vi "VisualizePmuAnalysis.vi"() -> ()   [LabVIEW 2018, in "Visualization.lvlib" / "VisualizeAnalysis.lvclass"]
uses:
  VisualizeAnalysis.lvclass
  <vilib>/event_ctls.llb/usereventprio.ctl
  VisualizeBase/VisualizeBase_class/Requests/clUserEventType.ctl
  <extravilib>/ChannelInstances/Tag-bool/Write With Abort.vi
  <extravilib>/ChannelInstances/Tag-bool/Read With Abort.vi
  <extravilib>/ChannelInstances/Tag-bool/Instantiate.vi
  <vilib>/Utility/error.llb/Error Cluster From Error Code.vi
  <extravilib>/ChannelInstances/Tag-bool/Endpoint.vi
  <vilib>/Utility/file.llb/Read From Spreadsheet File (DBL).vi
  <extravilib>/ChannelInstances/Tag-bool/EndpointRead.vi
  <vilib>/ErrorRing/Error Ring.xnode
  <userlib>/NIST/NISTErrorLib/NISTErrorLib.lvlib
  VisualizeBase/VisualizeBase_class/VisualizeBase.lvclass
  Analysis/AnalysisModule/AnalysisModule.lvlib
  VisualizeSensor/VisualizeSensor.lvclass
  <extravilib>/ChannelInstances/Tag-bool.lvlib
  TestClass/Test.lvclass
panel:
  in  "ModuleID":i32
  in  "btnClearTest":bool
  in  "btnReset":bool
  in  "btnPause":bool
  in  "btnOpen":bool
  in  "btnStop":bool
  in  "PluginName":string="Sensor.RoomAlert1"
  in  "Log Data":bool=TRUE
  out "Data from file":dbl[][](array[numeric])
  out "TVE":cluster{timestamp[], dbl[]}[](graph)
  out "FE":dbl(graph)=1.1347977483922023e-05
  out "ErrorArray":errorcluster[](array[cluster])
  out "RFE":dbl(graph)=-0.0019269131938461162
  out "Data real time":dbl[](array[numeric])
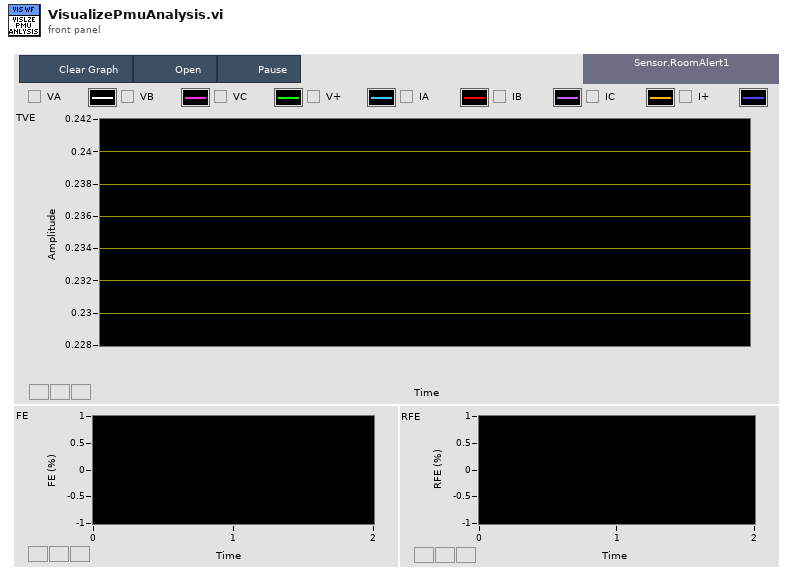
[diagram p1: front panel]
types:
  T1 = typedef "Visualization.lvlib/VisualizeBase.lvclass/clRequestEvents.ctl" = cluster{"StopRequest":refnum<user-event>, "ResetRequest":refnum<user-event>, "FP Pop In or Out":refnum<user-event>}
  T2 = typedef "AnalysisModule.lvlib/clBroadcastEvents.ctl" = cluster{"DidInit":refnum<user-event>, "StatusUpdate":refnum<user-event>, "ErrorReport":refnum<user-event>, "DidStop":refnum<user-event>, "PathToINI":refnum<user-event>, "Config":refnum<user-event>, "ResultReport":refnum<user-event>, "FunctionClass":refnum<user-event>, "State":refnum<user-event>, "FunctionParams":refnum<user-event>, "Duration":refnum<user-event>}
  T3 = enum16{"open", "open or create", "create or replace", "create", "open (read-only)"}
  T4 = typedef "Visualization.lvlib/VisualizeBase.lvclass/clUserEventType.ctl" = cluster{"BusIndex":i8, "Data":variant}
  T5 = typedef "usereventprio.ctl" = enum32{"high priority", "normal priority"}
  T6 = typedef "Tag-bool.lvlib/))Channel.ctl" = refnum<queue>
  T7 = typedef "sizeaction.ctl" = enum32{"Minimized", "Maximized", "Resized"}
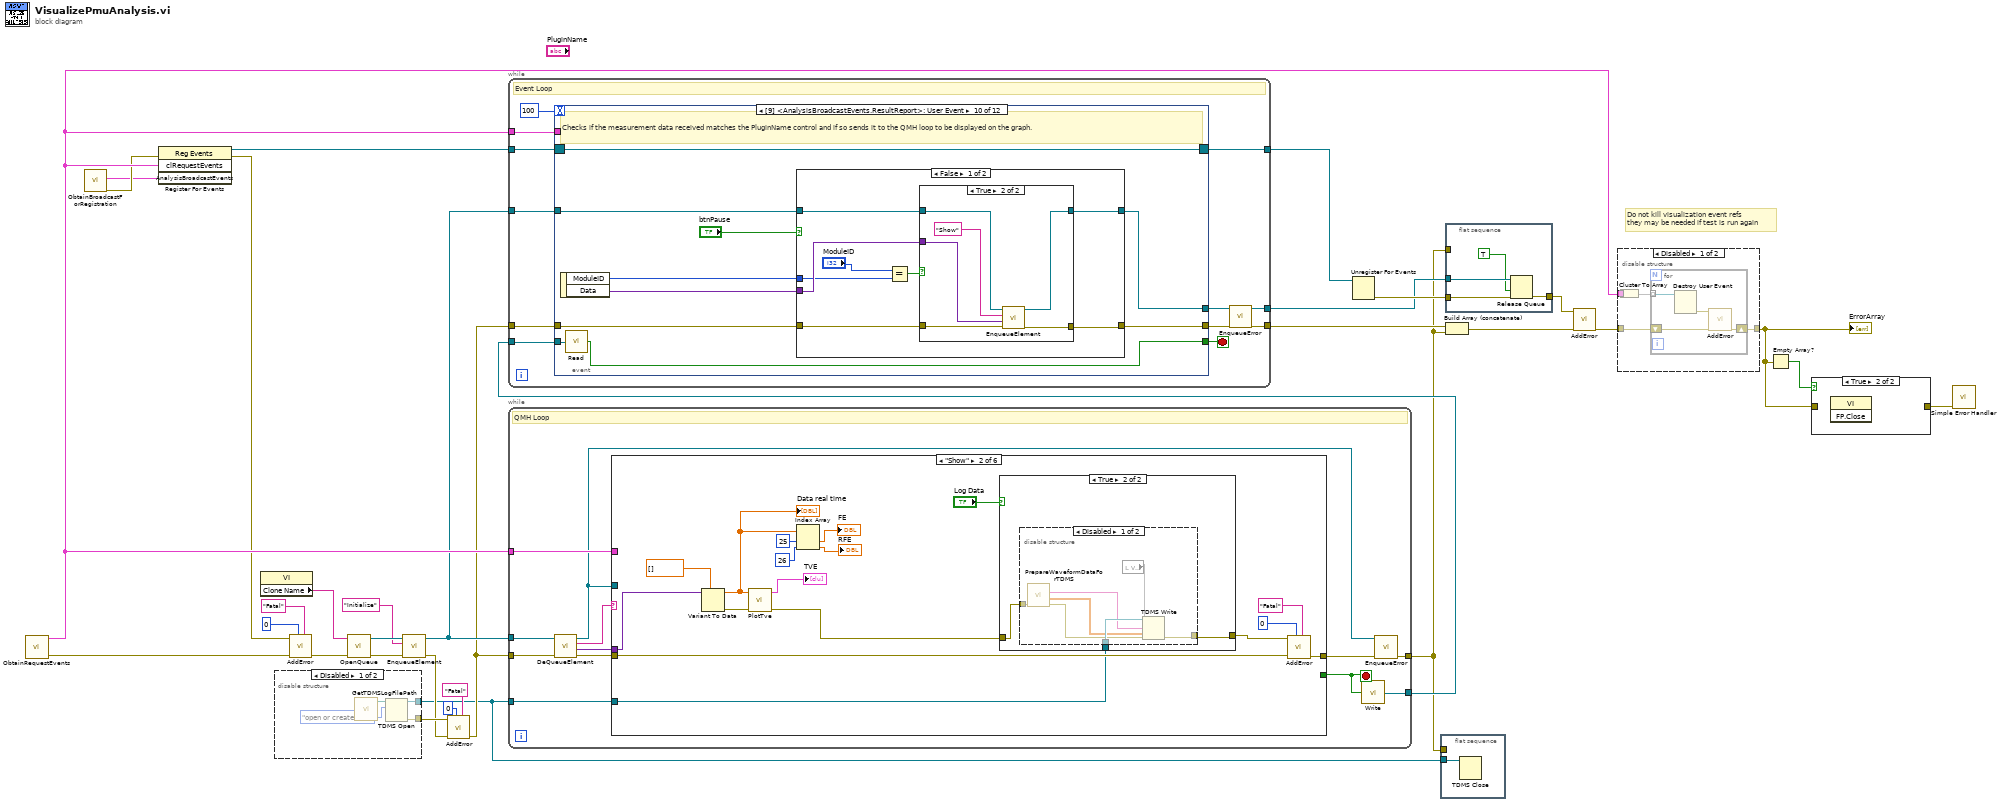
[diagram p0: block diagram]
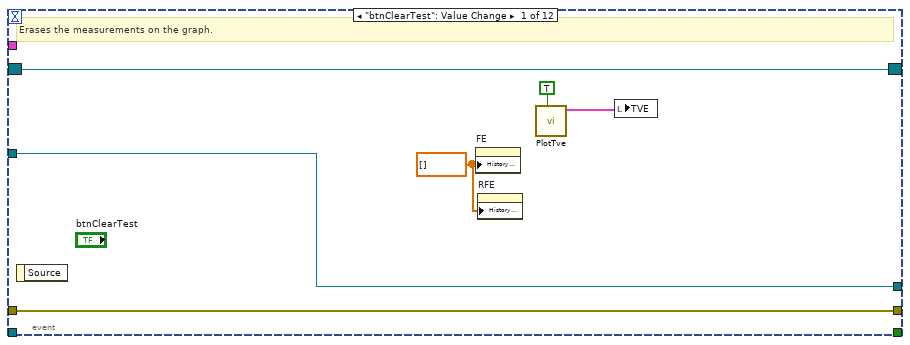
[diagram p4: hidden frame]
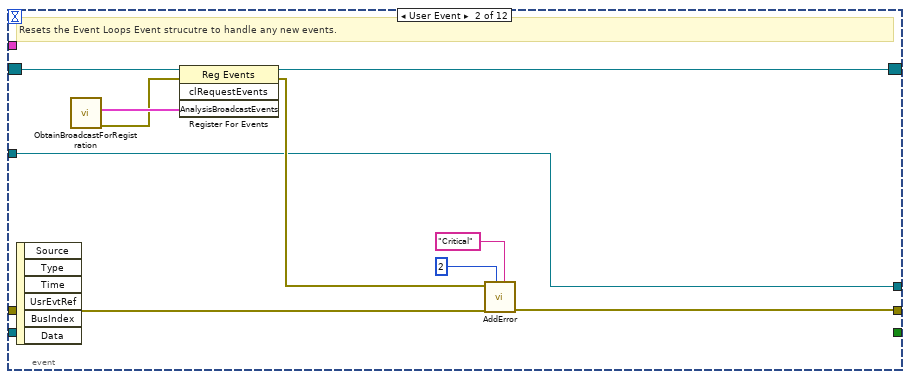
[diagram p5: hidden frame]
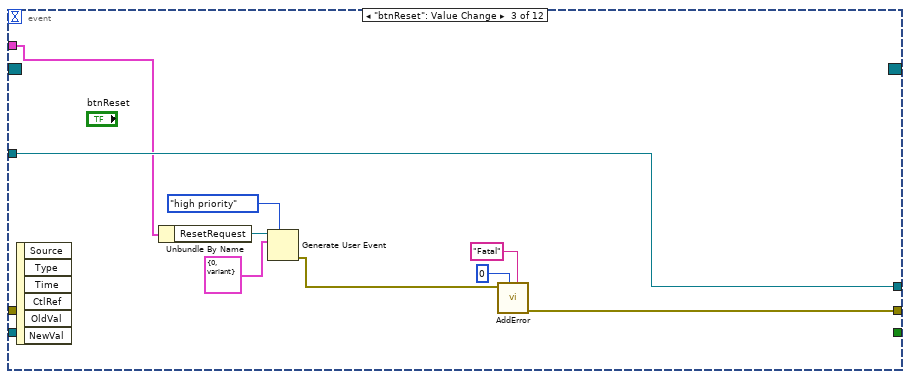
[diagram p6: hidden frame]
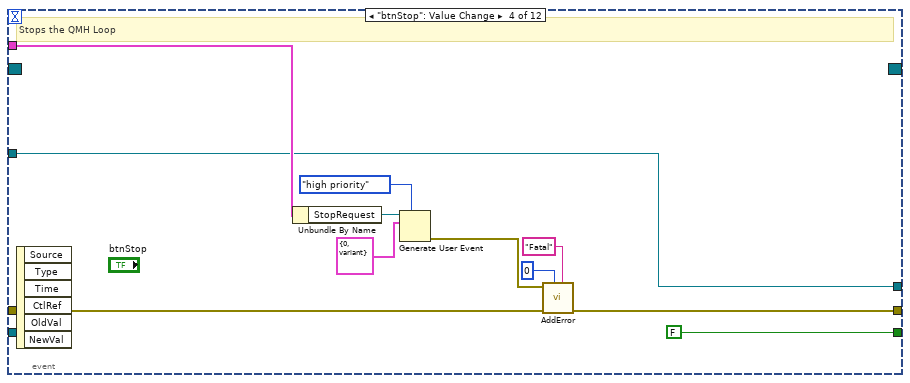
[diagram p7: hidden frame]
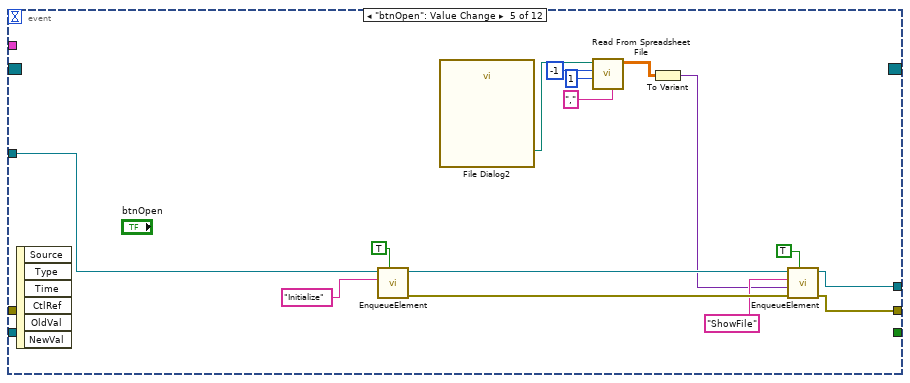
[diagram p8: hidden frame]
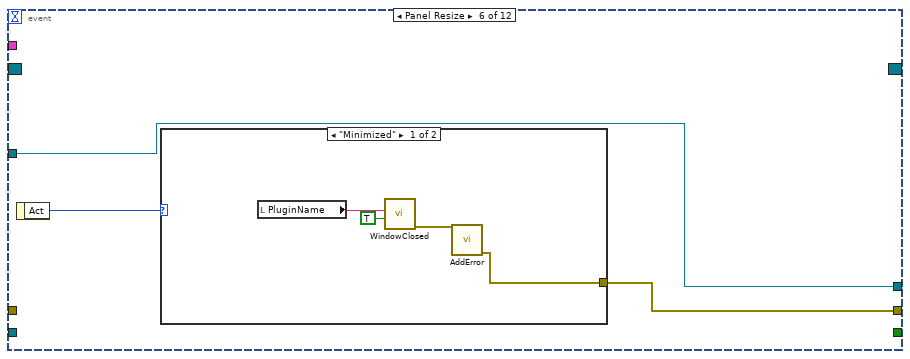
[diagram p9: hidden frame]
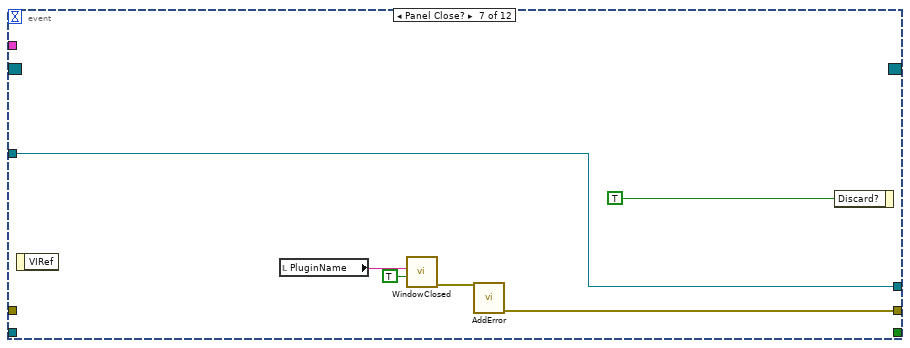
[diagram p11: hidden frame]
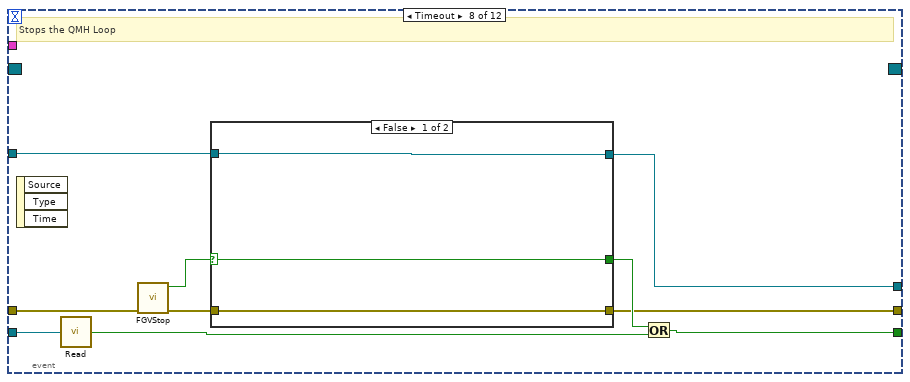
[diagram p12: hidden frame]
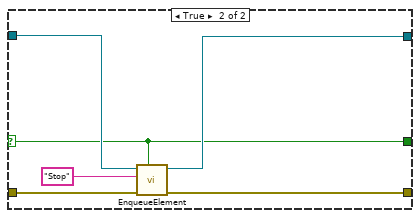
[diagram p13: hidden frame]
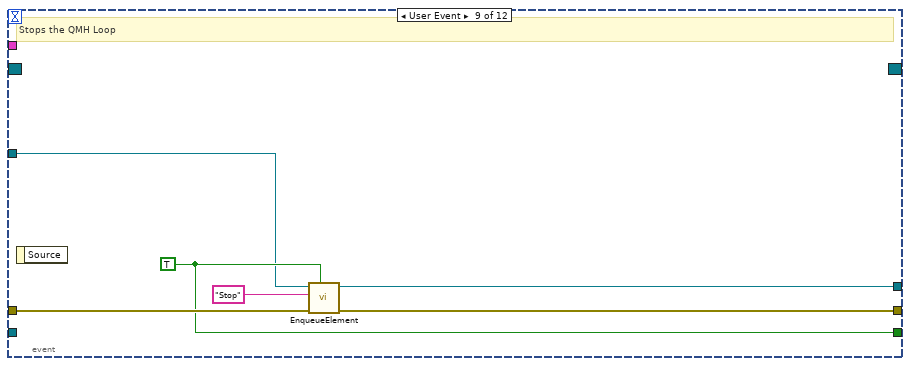
[diagram p14: hidden frame]
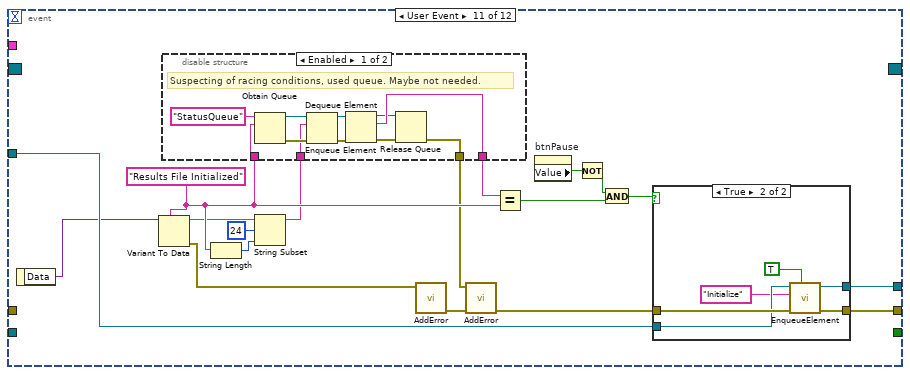
[diagram p17: hidden frame]
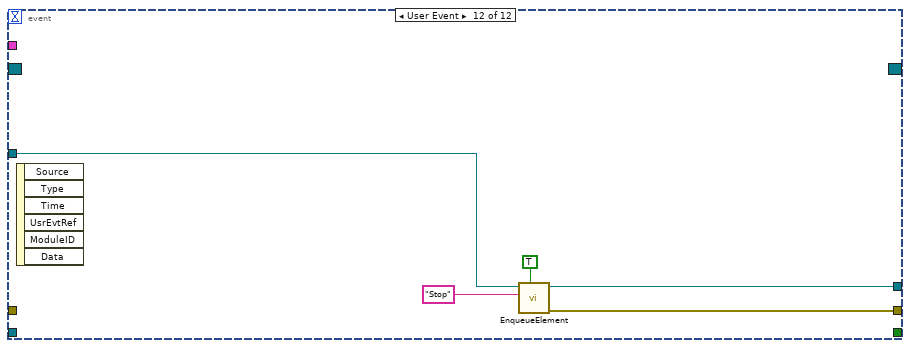
[diagram p20: hidden frame]
diagram:
  # "Do not kill visualization event refs\nthey may be needed if test is run again"
  n1 = call "ObtainRequestEvents.vi"() -> ("Error"=w23:errorcluster[], "clRequestEvents"=w25:T1)  [unwired: 10 in]
  n2 = call "ObtainBroadcastForRegistration.vi"() -> ("error out"=w3:errorcluster, "AnalysisBroadcastEvents"=w2:T2)  [unwired: 10 in]
  n3 = register-events(error in=w3, w25, w2) -> (reference out=w32:refnum<event-registration>, error out=w22:errorcluster)  [unwired: 1 in]
  n4 = property class="VI"() -> ("Clone Name"=w11:string)  [unwired: 2 in, 2 out]
  n5 = disable-structure shown="Disabled" {
    disable-tunnel: [w35 _] -> w8
    disable-tunnel: [w33 _] -> w5
    frame Disabled {
      n6 = call "GetTDMSLogFilePath.vi"() -> ("TDMS Log File Path"=w36:path)  [unwired: 11 in]
      n7 = TDMS Open(10:T3."open or create" ("operation (0:open)"), 11:w36) -> (0:w35:errorcluster, 3:w33:refnum<k34>)  [unwired: 5 in]
    }
    frame Enabled {
    }
  }
  n8 = call <userlib>:"AddError.vi"("Severity"="Fatal", "Priority"=u8 0, "ErrorArray In"=w23, "error in (no error)"=w22) -> ("ErrorArray Out"=w19:errorcluster[])  [unwired: 6 in, 1 out]
  n9 = call "OpenQueue.vi"("Error Array In"=w19, "QueueName"=w11) -> ("Error Array Out"=w17:errorcluster[], "queue out"=w18:refnum<queue>)  [unwired: 8 in]
  n10 = call "EnqueueElement.vi"("Error Array In"=w17, "Message"="Initialize", "queue in"=w18) -> ("Error Array Out"=w7:errorcluster[], "queue out"=w15:refnum<queue>)  [unwired: 7 in]
  n11 = call <userlib>:"AddError.vi"("Severity"="Fatal", "Priority"=u8 0, "ErrorArray In"=w7, "error in (no error)"=w8) -> ("ErrorArray Out"=w6:errorcluster[])  [unwired: 6 in, 1 out]
  n12 = while {
    tunnel: w6 -> [w42]
    tunnel: [w45] -> w4
    tunnel: w15 -> [w41]
    tunnel: w25 -> [w47]
    tunnel: [w38] -> w12
    tunnel: w5 -> [w37]
    stop <- w48 stop-if-true
    # "QMH Loop"
    n13 = call "DeQueueElement.vi"("Error Array In"=w42, "Queue In"=w41) -> ("Error Array Out"=w40:errorcluster[], "Data"=w43:variant, "Message"=w44:string, "Queue Out"=w39:refnum<queue>)  [unwired: 6 in]
    n14 = case shown="\"Show\"" w44 {
      selector: w44 -> [_ _ _ w104 _ _]
      tunnel: w43 -> [_ w53 w79 _ w123 _]
      tunnel: w40 -> [w50 w66 _ w102 _ w150]
      tunnel: [w50 w67 _ w101 w113 w150] -> w46
      tunnel: [_ _ _ _ w119 TRUE] -> w48
      tunnel: w47 -> [_ _ _ _ w118 _]
      tunnel: w39 -> [_ _ _ _ w117 _]
      tunnel: w37 -> [_ w61 _ _ _ _]
      frame "Initialize" {
        w49 = dbl[] [] ("History Data")
        (unwired) dbl[][] [] ("History Data")
        n15 = property on="FE" class="WFChart (strict)"("History Data"=w49) -> ()  [unwired: 2 in, 2 out]
        n16 = property on="RFE" class="WFChart (strict)"("History Data"=w49) -> ()  [unwired: 2 in, 2 out]
      }
      frame "Show" {
        n17 = Variant To Data(type=dbl[] [], Variant=w53) -> (data=w58:dbl[], error out=w51:errorcluster)  [unwired: 1 in]
        "Data real time" <- w58
        n18 = call "PlotTve.vi"("error in (no error)"=w51, "Data real time"=w58) -> ("error out"=w52:errorcluster, "TVE"=→"TVE":cluster{timestamp[], dbl[]}[])  [unwired: 8 in]
        n19 = Index Array(array=w58, index #1=25 ("index"), index #2=26 ("index")) -> (element #1=→"FE":dbl, element #2=→"RFE":dbl)
        n20 = case shown="True" "Log Data" {
          tunnel: w52 -> [w68 w70]
          tunnel: [w68 w71] -> w63
          tunnel: w61 -> [_ w69]
          frame False {
          }
          frame True {
            n21 = disable-structure shown="Disabled" {
              disable-tunnel: [w78 _] -> w71
              disable-tunnel: w70 -> [w77 _]
              disable-tunnel: w69 -> [w75 _]
              frame Disabled {
                n22 = call "PrepareWaveformDataForTDMS.vi"("error in (no error)"=w77) -> ("error out"=w74:errorcluster, "Measurement Data"=w72:dbl[][], "Channel Names"=w73:string[])  [unwired: 8 in]
                n23 = local read item#-1() -> (w76)
                n24 = TDMS Write(0:w75, 5:w76, 7:w73, 9:w72, 11:w74) -> (15:w78:errorcluster)  [unwired: 1 in, 3 out]
              }
              frame Enabled {
              }
            }
          }
        }
        n25 = call <userlib>:"AddError.vi"("Severity"="Fatal" ("String"), "Priority"=u8 0, "ErrorArray In"=w66, "error in (no error)"=w63) -> ("ErrorArray Out"=w67:errorcluster[])  [unwired: 6 in, 1 out]
      }
      frame "ShowFile" {
        n26 = Variant To Data(type=dbl[][] [], Variant=w79) -> (data=w92:dbl[][])  [unwired: 1 in, 1 out]
        "Data from file" <- w92
        n27 = Index Array(array=w92, index (col) #1=1 ("disabled index (col)"), index (col) #2=4 ("index (col)"), index (col) #3=7 ("index (col)"), index (col) #4=10 ("index (col)")) -> (element #1=w88:dbl[], element #2=w89:dbl[], element #3=w90:dbl[], element #4=w95:dbl[])  [unwired: 4 in]
        n28 = Index Array(array=w92, index (col) #1=25 ("disabled index (col)"), index (col) #2=26 ("index (col)")) -> (element #1=w93:dbl[], element #2=w94:dbl[])  [unwired: 2 in]
        n29 = Array Size(array=w95) -> (size(s)=w96:i32)
        n30 = Initialize Array(1.0 ("element"), w96) -> (w97:dbl[])
        n31 = property on="FE" class="WFChart (strict)"("History Data"=w93) -> ()  [unwired: 2 in, 2 out]
        n32 = Build Array(w88, w89, w90, w95, w97) -> (w91:dbl[][])
        n33 = property on="RFE" class="WFChart (strict)"("History Data"=w94) -> ()  [unwired: 2 in, 2 out]
        n34 = Transpose 2D Array(2D array=w91) -> ()  [unwired: 1 out]
      }
      frame Default {
        n35 = xnode "Error Ring"("parameter 0"=w104) -> ("error out"=w103:errorcluster)
        n36 = call <userlib>:"AddError.vi"("Severity"="Inform" ("String"), "Priority"=u8 5, "ErrorArray In"=w102, "error in (no error)"=w103) -> ("ErrorArray Out"=w101:errorcluster[], "error out"=w100:errorcluster)  [unwired: 6 in]
        n37 = call <vilib>:"Clear Errors.vi"("error in (no error)"=w100) -> ()  [unwired: 5 in, 2 out]
      }
      frame "Error" {
        n38 = Variant To Data(type=errorcluster[] [], Variant=w123) -> (data=w121:errorcluster[], error out=w112:errorcluster)  [unwired: 1 in]
        n39 = call <userlib>:"ParseErrors.vi"("ErrorArray"=w121) -> ("ErrorArray"=w120:errorcluster[])  [unwired: 8 in, 2 out]
        n40 = for {
          tunnel: w120 -> [w134] mode=indexing
          tunnel: [w128] -> w114 mode=concatenating
          tunnel: [w126] -> w119
          tunnel: w118 -> [w125]
          tunnel: w117 -> [w124]
          stop <- w126 stop-if-true
          n41 = call <userlib>:"GeneralHandler.vi"("error in (no error)"=w134) -> ("Severity"=w127:string, "Stop"=w131:bool, "Abort"=w132:bool, "Continue"=w133:bool)  [unwired: 6 in, 1 out]
          n42 = Build Array(w133, w132, w131) -> (w130:bool[])
          n43 = Boolean Array To Number(Boolean array=w130) -> (number=w129:u32)
          n44 = case shown="4" w129 {
            tunnel: [_ _ w139 w148] -> w128
            tunnel: w127 -> [_ _ _ w141]
            tunnel: [_ _ _ w143] -> w126
            tunnel: w125 -> [_ _ _ w142]
            tunnel: w124 -> [_ _ w135 _]
            frame 0, Default {
              # "No Dialog"
            }
            frame 1 {
              # "Continue"
            }
            frame 2 {
              # "Abort, Flush Queue"
              n45 = Flush Queue(queue=w135) -> (error out=w138:errorcluster)  [unwired: 1 in, 2 out]
              n46 = call <userlib>:"AddError.vi"("Severity"="Critical" ("String"), "Priority"=u8 1, "error in (no error)"=w138) -> ("ErrorArray Out"=w139:errorcluster[])  [unwired: 7 in, 1 out]
            }
            frame 4 {
              # "Stop"
              n47 = Unbundle By Name(w142) -> ("StopRequest"=w149:refnum<user-event>)
              n48 = Equal?(x=w141, y="Fatal" ("x")) -> (x = y?=w143:bool)
              n49 = Generate User Event(priority (normal)=usereventprio."high priority", user event=w149, event data cluster=T4 {"BusIndex"=0, "Data"=variant} ("event data")) -> (error out=w147:errorcluster)  [unwired: 1 in, 1 out]
              n50 = call <userlib>:"AddError.vi"("error in (no error)"=w147) -> ("ErrorArray Out"=w148:errorcluster[], "error out"=w144:errorcluster)  [unwired: 9 in]
              n51 = call <vilib>:"Clear Errors.vi"("error in (no error)"=w144) -> ()  [unwired: 5 in, 2 out]
            }
          }
        }
        n52 = call <userlib>:"AddError.vi"("Severity"="Critical", "Priority"=u8 2, "ErrorArray In"=w114, "error in (no error)"=w112) -> ("ErrorArray Out"=w113:errorcluster[])  [unwired: 6 in, 1 out]
      }
      frame "Stop" {
      }
    }
    n53 = call <extravilib>:"Write.vi"("element"=w48) -> ("channel"=w38:T6)  [unwired: 1 out]
    n54 = call "EnqueueError.vi"("Error Array In"=w46, "Queue in"=w39) -> ("Error Array Out"=w45:errorcluster[])  [unwired: 8 in, 1 out]
  }
  n55 = while {
    tunnel: w32 -> [w163]
    tunnel: [w157] -> w30
    tunnel: [w161] -> w31
    tunnel: w25 -> [w160]
    tunnel: w6 -> [w159]
    tunnel: w15 -> [w158]
    tunnel: [w154] -> w14
    tunnel: w12 -> [w152]
    stop <- w162 stop-if-true
    # "Event Loop"
    n56 = event shown="[9] <AnalysisBroadcastEvents.ResultReport>: User Event" {
      selector: w163 -> [w168 w179 _ _ _ _ _ _ _ w258 _ _]
      dyn-events: [w168 w178 _ _ _ _ _ _ _ w258 _ _] -> w161
      timeout: 100 -> [_ _ _ _ _ _ _ _ _ _ _ _]
      tunnel: [_ _ _ FALSE ("Priority? (F)") _ _ _ w228 w249 w255 _ _] -> w162
      tunnel: [w169 w176 w182 w192 w201 w216 w222 w230 w251 w260 w283 w321] -> w156
      tunnel: w160 -> [_ _ w180 w191 _ _ _ _ _ _ _ _]
      tunnel: w159 -> [w169 w177 _ w199 _ _ _ w233 w252 w261 _ _]
      tunnel: w158 -> [w167 w172 w181 w189 w209 w215 w226 w232 w247 w262 w285 w319]
      tunnel: [w167 w172 w181 w189 w200 w215 w226 w231 w250 w259 w282 w320] -> w155
      tunnel: w152 -> [_ _ _ _ _ _ _ w237 _ w256 _ _]
      event "btnClearTest": Value Change {
        w166 = dbl[] [] ("History Data")
        # "Erases the measurements on the graph."
        n57 = event-data() -> ()  [unwired: 1 in, 1 out]
        n58 = property on="FE" class="WFChart (strict)"("History Data"=w166) -> ()  [unwired: 2 in, 2 out]
        n59 = property on="RFE" class="WFChart (strict)"("History Data"=w166) -> ()  [unwired: 2 in, 2 out]
        n60 = call "PlotTve.vi"("Clear? (f)"=TRUE) -> ("TVE"=w165:cluster{timestamp[], dbl[]}[])  [unwired: 9 in, 1 out]
        n61 = local write "TVE"(w165) -> ()
      }
      event User Event {
        # "Resets the Event Loops Event strucutre to handle any new events."
        n62 = event-data() -> ()  [unwired: 1 in, 6 out]
        n63 = call "ObtainBroadcastForRegistration.vi"() -> ("error out"=w170:errorcluster, "AnalysisBroadcastEvents"=w171:T2)  [unwired: 10 in]
        n64 = register-events(reference=w179, error in=w170, w171) -> (reference out=w178:refnum<event-registration>, error out=w173:errorcluster)  [unwired: 1 in]
        n65 = call <userlib>:"AddError.vi"("Severity"="Critical", "Priority"=u8 2, "ErrorArray In"=w177, "error in (no error)"=w173) -> ("ErrorArray Out"=w176:errorcluster[])  [unwired: 6 in, 1 out]
      }
      event "btnReset": Value Change {
        n66 = event-data() -> ()  [unwired: 1 in, 6 out]
        n67 = Unbundle By Name(w180) -> ("ResetRequest"=w188:refnum<user-event>)
        n68 = Generate User Event(priority (normal)=usereventprio."high priority", user event=w188, event data cluster=T4 {"BusIndex"=0, "Data"=variant} ("event data")) -> (error out=w185:errorcluster)  [unwired: 1 in, 1 out]
        n69 = call <userlib>:"AddError.vi"("Severity"="Fatal", "Priority"=u8 0, "error in (no error)"=w185) -> ("ErrorArray Out"=w182:errorcluster[])  [unwired: 7 in, 1 out]
      }
      event "btnStop": Value Change {
        # "Stops the QMH Loop"
        n70 = event-data() -> ()  [unwired: 1 in, 6 out]
        n71 = Unbundle By Name(w191) -> ("StopRequest"=w197:refnum<user-event>)
        n72 = Generate User Event(priority (normal)=usereventprio."high priority", user event=w197, event data cluster=T4 {"BusIndex"=0, "Data"=variant} ("event data")) -> (error out=w198:errorcluster)  [unwired: 1 in, 1 out]
        n73 = call <userlib>:"AddError.vi"("Severity"="Fatal" ("String"), "Priority"=u8 0, "ErrorArray In"=w199, "error in (no error)"=w198) -> ("ErrorArray Out"=w192:errorcluster[])  [unwired: 6 in, 1 out]
      }
      event "btnOpen": Value Change {
        n74 = event-data() -> ()  [unwired: 1 in, 6 out]
        n75 = call "EnqueueElement.vi"("Priority? (F)"=TRUE, "Message"="Initialize", "queue in"=w209) -> ("Error Array Out"=w205:errorcluster[], "queue out"=w203:refnum<queue>)  [unwired: 7 in]
        n76 = call "File Dialog2"() -> ("selected path"=w210:path)  [unwired: 12 in, 3 out]
        n77 = call-poly <vilib>:"Read From Spreadsheet File.vi"("delimiter (\\t)"="," ("delimiter (\\t)"), "start of read offset (chars.:0)"=1, "number of rows (all:-1)"=-1, "file path (dialog if empty)"=w210) -> ("all rows"=w212:dbl[][])  [unwired: 3 in, 4 out]
        n78 = To Variant(anything=w212) -> (Variant=w202:variant)
        n79 = call "EnqueueElement.vi"("Priority? (F)"=TRUE, "Error Array In"=w205, "Data"=w202, "Message"="ShowFile", "queue in"=w203) -> ("Error Array Out"=w201:errorcluster[], "queue out"=w200:refnum<queue>)  [unwired: 5 in]
      }
      event Panel Resize {
        n80 = event-data() -> ("Act"=w217:T7)  [unwired: 1 in]
        n81 = case shown="\"Minimized\"" w217 {
          tunnel: [w218 _] -> w216
          frame "Minimized" {
            n82 = local read "PluginName"() -> (w220:string)
            n83 = call "WindowClosed.vi"("Window Closed?"=TRUE ("Window Minimized or Clozed?"), "Module Name"=w220) -> ("error out"=w221:errorcluster)  [unwired: 9 in]
            n84 = call <userlib>:"AddError.vi"("error in (no error)"=w221) -> ("ErrorArray Out"=w218:errorcluster[])  [unwired: 9 in, 1 out]
          }
          frame "Maximized", Default {
          }
        }
      }
      event Panel Close? {
        n85 = event-data() -> ()  [unwired: 1 in, 1 out]
        n86 = local read "PluginName"() -> (w223:string)
        n87 = call "WindowClosed.vi"("Window Closed?"=TRUE ("Window Minimized or Clozed?"), "Module Name"=w223) -> ("error out"=w225:errorcluster)  [unwired: 9 in]
        n88 = call <userlib>:"AddError.vi"("error in (no error)"=w225) -> ("ErrorArray Out"=w222:errorcluster[])  [unwired: 9 in, 1 out]
        n89 = event-data("Discard?"=TRUE) -> ()  [unwired: 1 in, 1 out]
      }
      event Timeout {
        # "Stops the QMH Loop"
        n90 = event-data() -> ()  [unwired: 1 in, 3 out]
        n91 = call <extravilib>:"Read.vi"("channel"=w237) -> ("element"=w229:bool)  [unwired: 1 in, 1 out]
        n92 = call "FGVStop.vi"("Error In"=w233) -> ("Error Out"=w235:errorcluster[], "Value"=w236:bool)  [unwired: 9 in]
        n93 = case shown="False" w236 {
          selector: w236 -> [w238 w241]
          tunnel: [w240 w244] -> w230
          tunnel: w235 -> [w240 w245]
          tunnel: w232 -> [w239 w243]
          tunnel: [w239 w242] -> w231
          tunnel: [w238 w241] -> w234
          frame False {
          }
          frame True {
            n94 = call "EnqueueElement.vi"("Priority? (F)"=w241, "Error Array In"=w245, "Message"="Stop", "queue in"=w243) -> ("Error Array Out"=w244:errorcluster[], "queue out"=w242:refnum<queue>)  [unwired: 6 in]
          }
        }
        n95 = Or(x=w234, y=w229) -> (x .or. y?=w228:bool)
      }
      event User Event {
        w249 = TRUE ("Priority? (F)")
        # "Stops the QMH Loop"
        n96 = event-data() -> ()  [unwired: 1 in, 1 out]
        n97 = call "EnqueueElement.vi"("Priority? (F)"=w249, "Error Array In"=w252, "Message"="Stop", "queue in"=w247) -> ("Error Array Out"=w251:errorcluster[], "queue out"=w250:refnum<queue>)  [unwired: 6 in]
      }
      event User Event {
        # "Checks if the measurement data received matches the PluginName control and if so sends it to the QMH loop to be displayed on the graph."
        n98 = event-data() -> ("ModuleID"=w253:i32, "Data"=w257:variant)  [unwired: 1 in]
        n99 = call <extravilib>:"Read.vi"("channel"=w256) -> ("element"=w255:bool)  [unwired: 1 in, 1 out]
        n100 = case shown="False" "btnPause" {
          tunnel: w262 -> [w270 w280]
          tunnel: w261 -> [w269 w279]
          tunnel: [w263 w279] -> w260
          tunnel: [w268 w280] -> w259
          tunnel: w257 -> [w267 _]
          tunnel: w253 -> [w266 _]
          frame False {
            n101 = Equal?(x="ModuleID", y=w266) -> (x = y?=w265:bool)
            n102 = case shown="True" w265 {
              tunnel: [w271 w277] -> w263
              tunnel: w270 -> [w272 w276]
              tunnel: w269 -> [w271 w278]
              tunnel: [w272 w274] -> w268
              tunnel: w267 -> [_ w275]
              frame False {
              }
              frame True {
                n103 = call "EnqueueElement.vi"("Error Array In"=w278, "Data"=w275, "Message"="Show", "queue in"=w276) -> ("Error Array Out"=w277:errorcluster[], "queue out"=w274:refnum<queue>)  [unwired: 6 in]
              }
            }
          }
          frame True {
          }
        }
      }
      event User Event {
        w295 = "Results File Initialized" ("Status")
        n104 = event-data() -> ("Data"=w284:variant)  [unwired: 1 in]
        n105 = Variant To Data(type=w295, Variant=w284) -> (data=w287:string, error out=w290:errorcluster)  [unwired: 1 in]
        n106 = String Length(string=w295) -> (length=w294:i32)
        n107 = String Subset(string=w287, offset (0)=24, length (rest)=w294) -> (substring=w292:string)
        n108 = disable-structure shown="Enabled" {
          disable-tunnel: [w302 w310] -> w288
          disable-tunnel: [w299 _] -> w291
          disable-tunnel: w292 -> [w304 w310]
          disable-tunnel: w295 -> [w303 _]
          frame Enabled {
            # "Suspecting of racing conditions, used queue. Maybe not needed."
            n109 = Obtain Queue(name (unnamed)="StatusQueue", element data type=w303) -> (queue out=w308:refnum<queue>, error out=w306:errorcluster)  [unwired: 3 in, 1 out]
            n110 = Enqueue Element(queue=w308, element=w304, error in (no error)=w306) -> (queue out=w307:refnum<queue>, error out=w305:errorcluster)  [unwired: 1 in, 1 out]
            n111 = Dequeue Element(queue=w307, error in (no error)=w305) -> (queue out=w301:refnum<queue>, element=w302:string, error out=w300:errorcluster)  [unwired: 1 in, 1 out]
            n112 = Release Queue(queue=w301, error in (no error)=w300) -> (error out=w299:errorcluster)  [unwired: 1 in, 2 out]
          }
          frame Disabled {
          }
        }
        n113 = call <userlib>:"AddError.vi"("error in (no error)"=w290) -> ("ErrorArray Out"=w289:errorcluster[])  [unwired: 9 in, 1 out]
        n114 = call <userlib>:"AddError.vi"("ErrorArray In"=w289, "error in (no error)"=w291) -> ("ErrorArray Out"=w286:errorcluster[])  [unwired: 8 in, 1 out]
        n115 = Equal?(x=w288, y=w295) -> (x = y?=w296:bool)
        n116 = property on="btnPause" class="Bool (strict)"() -> ("Value"=w297:bool)  [unwired: 2 in, 2 out]
        n117 = Not(x=w297) -> (.not. x?=w298:bool)
        n118 = And(x=w298, y=w296) -> (x .and. y?=w281:bool)
        n119 = case shown="True" w281 {
          tunnel: [w312 w317] -> w283
          tunnel: w286 -> [w312 w318]
          tunnel: w285 -> [w311 w316]
          tunnel: [w311 w313] -> w282
          frame False {
          }
          frame True {
            n120 = call "EnqueueElement.vi"("Priority? (F)"=TRUE, "Error Array In"=w318, "Message"="Initialize", "queue in"=w316) -> ("Error Array Out"=w317:errorcluster[], "queue out"=w313:refnum<queue>)  [unwired: 6 in]
          }
        }
      }
      event User Event {
        n121 = event-data() -> ()  [unwired: 1 in, 6 out]
        n122 = call "EnqueueElement.vi"("Priority? (F)"=TRUE, "Message"="Stop", "queue in"=w319) -> ("Error Array Out"=w321:errorcluster[], "queue out"=w320:refnum<queue>)  [unwired: 7 in]
      }
    }
    n123 = call "EnqueueError.vi"("Error Array In"=w156, "Queue in"=w155) -> ("Error Array Out"=w157:errorcluster[], "Queue out"=w154:refnum<queue>)  [unwired: 8 in]
  }
  n124 = Unregister For Events(event registration refnum=w31) -> (error out=w29:errorcluster)  [unwired: 1 in]
  n125 = flat-sequence {
    tunnel: w5 -> [w324]
    tunnel: w4 -> [_]
    frame #0 {
      n126 = TDMS Close(11:w324) -> ()  [unwired: 1 in, 2 out]
    }
  }
  n127 = flat-sequence {
    tunnel: w29 -> [w328]
    tunnel: [w327] -> w27
    tunnel: w14 -> [w326]
    tunnel: w4 -> [_]
    frame #0 {
      n128 = Release Queue(queue=w326, force destroy? (F)=TRUE, error in (no error)=w328) -> (error out=w327:errorcluster)  [unwired: 2 out]
    }
  }
  n129 = Build Array (concatenate)(w30, w4) -> (w28:errorcluster[])
  n130 = call <userlib>:"AddError.vi"("ErrorArray In"=w28, "error in (no error)"=w27) -> ("ErrorArray Out"=w26:errorcluster[])  [unwired: 8 in, 1 out]
  n131 = disable-structure shown="Disabled" {
    disable-tunnel: w26 -> [w331 w337]
    disable-tunnel: w25 -> [w330 _]
    disable-tunnel: [w329 w337] -> w1
    frame Disabled {
      n132 = Cluster To Array(cluster=w330) -> (array=w332:refnum<user-event>[])
      n133 = for {
        tunnel: w332 -> [w336] mode=indexing
        shift-right: [w335] -> w329
        shift-left: w331 -> [w334]
        n134 = Destroy User Event(user event=w336) -> (error out=w333:errorcluster)  [unwired: 1 in]
        n135 = call <userlib>:"AddError.vi"("ErrorArray In"=w334, "error in (no error)"=w333) -> ("ErrorArray Out"=w335:errorcluster[])  [unwired: 8 in, 1 out]
      }
    }
    frame Enabled {
    }
  }
  "ErrorArray" <- w1
  n136 = Empty Array?(array=w1) -> (empty?=w24:bool)
  n137 = case shown="True" w24 {
    tunnel: [w338 _] -> w13
    tunnel: w1 -> [w339 _]
    frame False {
      n138 = Merge Errors(w339) -> (w338:errorcluster)
    }
    frame True {
      n139 = invoke class="VI" method="FP.Close"() -> ()  [unwired: 3 in, 3 out]
    }
  }
  n140 = call <vilib>:"Simple Error Handler.vi"("error in (no error)"=w13) -> ()  [unwired: 4 in, 5 out]
